vi "Interface Write N Start Time.vi"(7 "count (1)":i32=1, 8 "error in (no error)":errorcluster, 11 "Dispatcher Interface in":refnum<class "Dispatcher Interface.lvclass">) -> (0 "error out":errorcluster, 3 "Dispatcher Interface out":refnum<class "Dispatcher Interface.lvclass">)   [LabVIEW 2017]
uses:
  Classes/Interfaces/Dispatcher/Dispatcher Interface.lvclass
  C:/Git/DSF/Data Sharing Framework/Source/Core/Engine/Classes/Interfaces/Interface/Interface.lvclass
  Classes/Interfaces/Dispatcher/Command Data.ctl
  Classes/Interfaces/Dispatcher/Command.ctl
  Classes/Interfaces/Dispatcher/Parameters.ctl
  Classes/Interfaces/Interface/Interface.lvclass/Interface.ctl
  Classes/Debug/FIFO Flags/FIFO Flags.lvclass/FIFO Flags.ctl
  Classes/Interfaces/Interface/Write Command.vi
  Classes/Interfaces/Interface/Get Command FIFO.vi
  Classes/Interfaces/Interface/Write RT FIFO(16B).vi
  Classes/Interfaces/Interface/Get Debug Flags.vi
  Classes/Debug/FIFO Flags/Get Infinite Timeouts.vi
  Classes/Interfaces/Interface/Errors.vi
  Classes/Interfaces/Interface/Command Timeout.vi
  Classes/Interfaces/Dispatcher/Write Dispatcher Command.vi
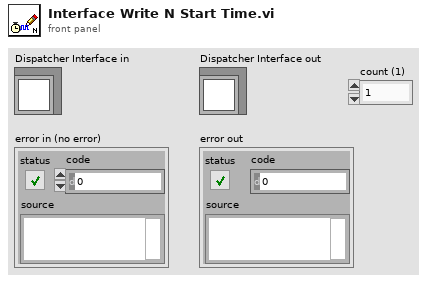
[diagram p1: front panel]
types:
  T1 = typedef "DSF Core.lvlib/Dispatcher Interface.lvclass/Command Data.ctl" = cluster{"Command":T2, "Parameters":T3}
  T2 = typedef "DSF Core.lvlib/Dispatcher Interface.lvclass/Command.ctl" = enum8{"Rx", "Tx", "Shutdown"}
  T3 = typedef "DSF Core.lvlib/Dispatcher Interface.lvclass/Parameters.ctl" = cluster{"arg1":u64, "arg2":u64}
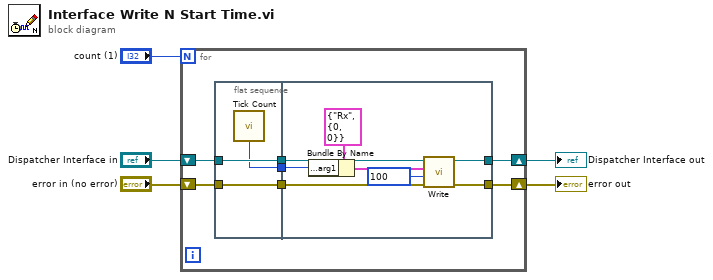
[diagram p0: block diagram]
diagram:
  n1 = for {
    N: "count (1)" -> [_]
    shift-right: [w10] -> w1
    shift-left: "Dispatcher Interface in" -> [w11]
    shift-right: [w9] -> w3
    shift-left: "error in (no error)" -> [w12]
    n2 = flat-sequence {
      tunnel: w11 -> [w14]
      tunnel: w12 -> [w15]
      tunnel: [w15] -> w8
      tunnel: [w14] -> w7
      tunnel: [w13] -> w6
      tunnel: [w21] -> w10
      tunnel: [w20] -> w9
      tunnel: w8 -> [w23]
      tunnel: w7 -> [w22]
      tunnel: w6 -> [w16]
      frame #0 {
        n3 = call "Tick Count"() -> ("Tick Count(uSec)"=w13:u32)
      }
      frame #1 {
        n4 = Bundle By Name(cluster=T1 {"Command"=enum."Rx", "Parameters"={"arg1"=0, "arg2"=0}} ("command"), "Parameters.arg1"=w16) -> (w17:T1)
        n5 = call-poly "Write.vi"("error in (no error)"=w23, "timeout in ms (0)"=100, "command"=w17, "Dispatcher Interface in"=w22) -> ("error out"=w20:errorcluster, "Dispatcher Interface out"=w21:refnum<class "Dispatcher Interface.lvclass">)  [unwired: 5 in, 1 out]
      }
    }
  }
  "error out" <- w3
  "Dispatcher Interface out" <- w1
